vi "MoveAxesAbsolute.vi"() -> ()   [LabVIEW 2015]
uses:
  <userlib>/Newport ESP301/Newport ESP301.lvlib
panel:
  in  "Position":dbl format="%#_13g"
  in  "Position":dbl format="%#_13g"
  in  "Position":dbl format="%#_13g"
  in  "Axis 3":bool
  in  "Axis 2":bool
  in  "Axis 1":bool
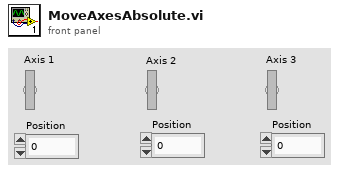
[diagram p1: front panel]
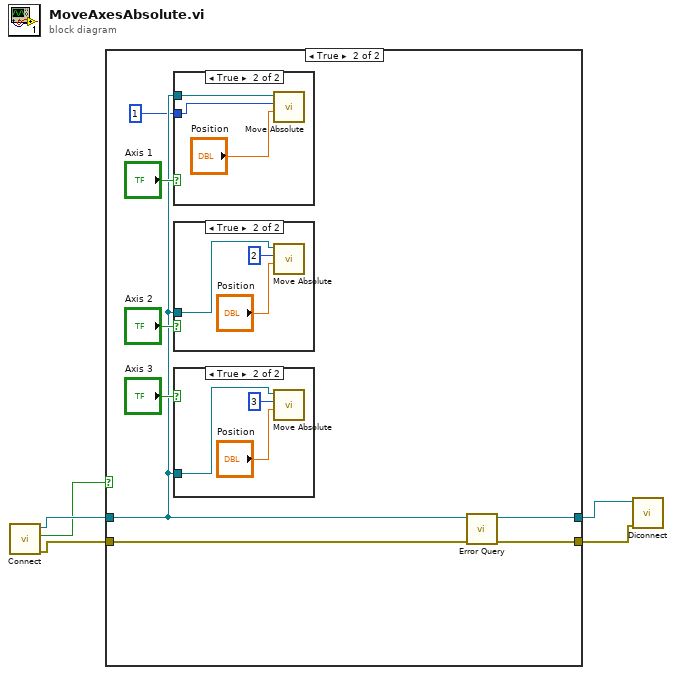
[diagram p0: block diagram]
diagram:
  n1 = call "Connect.vi"() -> ("error out"=w4:errorcluster, "Connected"=w3:bool, "VISA resource name out"=w5:refnum<visa-resource-name>)  [unwired: 5 in]
  n2 = case shown="True" w3 {
    tunnel: w5 -> [w7 w9]
    tunnel: w4 -> [w6 w12]
    tunnel: [w7 w10] -> w2
    tunnel: [w6 w11] -> w1
    frame False {
    }
    frame True {
      n3 = case shown="True" "Axis 1" {
        tunnel: w9 -> [_ w24]
        tunnel: 1 -> [_ w22]
        frame False {
        }
        frame True {
          n4 = call <userlib>:"Move Absolute.vi"("Position (0 units)"="Position", "Axis (1)"=w22, "VISA resource name"=w24) -> ()  [unwired: 3 in, 2 out]
        }
      }
      n5 = case shown="True" "Axis 2" {
        tunnel: w9 -> [_ w20]
        frame False {
        }
        frame True {
          n6 = call <userlib>:"Move Absolute.vi"("Position (0 units)"="Position", "Axis (1)"=2, "VISA resource name"=w20) -> ()  [unwired: 3 in, 2 out]
        }
      }
      n7 = case shown="True" "Axis 3" {
        tunnel: w9 -> [_ w16]
        frame False {
        }
        frame True {
          n8 = call <userlib>:"Move Absolute.vi"("Position (0 units)"="Position", "Axis (1)"=3, "VISA resource name"=w16) -> ()  [unwired: 3 in, 2 out]
        }
      }
      n9 = call <userlib>:"Error Query.vi"("error in (no error)"=w12, "VISA resource name"=w9) -> ("error out"=w11:errorcluster, "VISA resource name out"=w10:refnum<visa-resource-name>)  [unwired: 2 in, 2 out]
    }
  }
  n10 = call "Diconnect.vi"("error in (no error)"=w1, "VISA resource name"=w2) -> ()  [unwired: 6 in]
